vi "Display (SubVI).vi"(10 "Numeric 2":i32, 11 "Numeric":dbl) -> (1 "Formatted Array":u8[](array[numeric]), 3 "Formatted String":string)   [LabVIEW 2021]
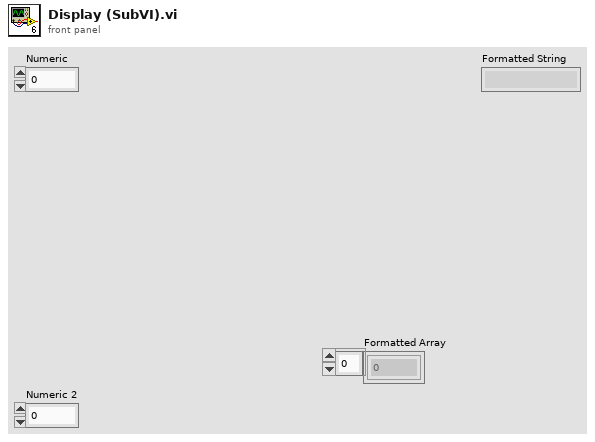
[diagram p1: front panel]
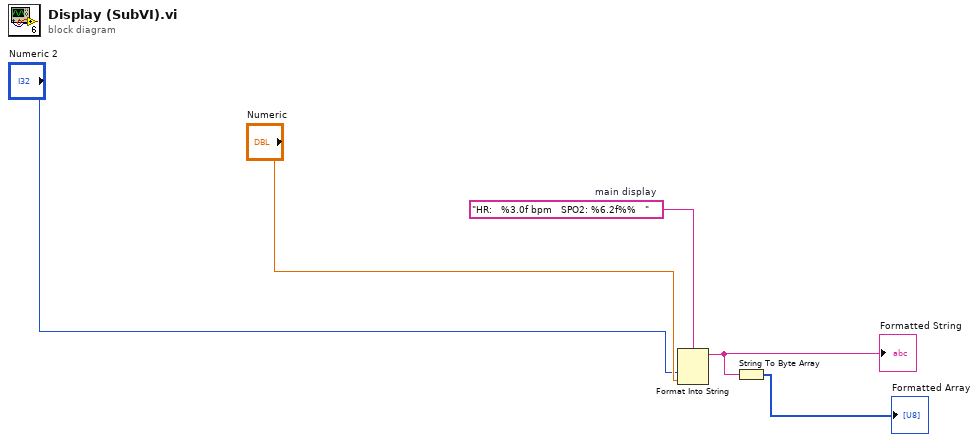
[diagram p0: block diagram]
diagram:
  w1 = "HR:   %3.0f bpm   SPO2: %6.2f%%   "  # main display
  n1 = Format Into String(format string=w1, "Numeric 2", "Numeric") -> (resulting string=w3:string)  [unwired: 2 in, 1 out]
  "Formatted String" <- w3
  n2 = String To Byte Array(string=w3) -> (unsigned byte array=→"Formatted Array":u8[])
